vi "Duplicate Targets.vi"(9 "Array":T1[](array[typedef])) -> (2 "Duplicates found":bool)   [LabVIEW 2009]
uses:
  MixedMode/Messages/Target.ctl
  Data Access Objects/Metadata/LBCB Number.ctl
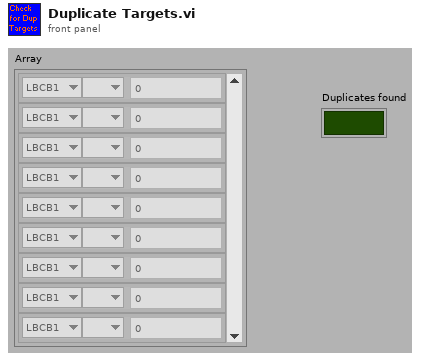
[diagram p1: front panel]
types:
  T1 = typedef "Target.ctl" = cluster{"LBCB Number":T2, "DOF Vectors":enum16{" ", "Dx", "Dy", "Dz", "Rx", "Ry", "Rz", "Fx", "Fy", "Fz", "Mx", "My", "Mz"}, "Amount":dbl}
  T2 = typedef "LBCB Number.ctl" = enum16{"LBCB1", "LBCB2"}
  T3 = enum16{" ", "Dx", "Dy", "Dz", "Rx", "Ry", "Rz", "Fx", "Fy", "Fz", "Mx", "My", "Mz"}
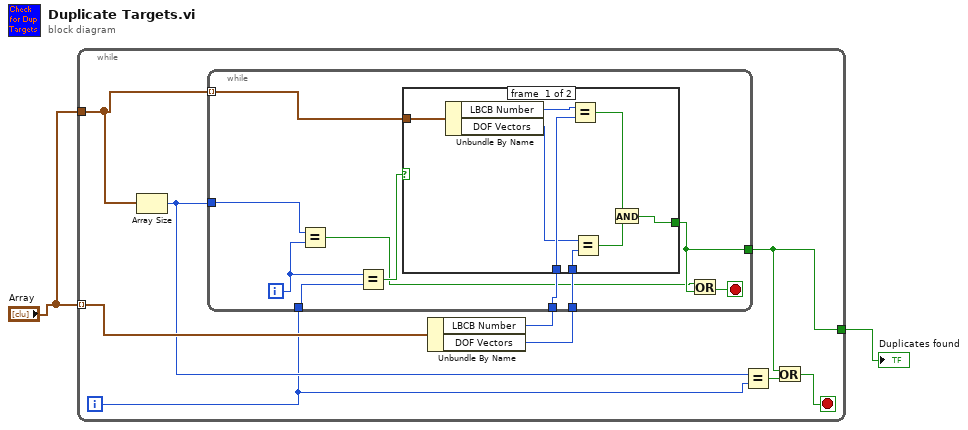
[diagram p0: block diagram]
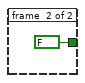
[diagram p2: hidden frame]
diagram:
  n1 = while {
    tunnel: "Array" -> [w9] mode=indexing
    tunnel: "Array" -> [w8]
    tunnel: [w4] -> w1
    i -> [w6]
    stop <- w3 stop-if-true
    n2 = Array Size(array=w8) -> (size(s)=w7:i32)
    n3 = Unbundle By Name(w9) -> ("LBCB Number"=w11:T2, "DOF Vectors"=w10:T3)
    n4 = while {
      tunnel: w11 -> [w21]
      tunnel: w10 -> [w20]
      tunnel: w8 -> [w19] mode=indexing
      tunnel: w6 -> [w18]
      tunnel: [w16] -> w4
      tunnel: w7 -> [w15]
      i -> [w14]
      stop <- w13 stop-if-true
      n5 = Equal?(x=w15, y=w14) -> (x = y?=w12:bool)
      n6 = Equal?(x=w14, y=w18) -> (x = y?=w17:bool)
      n7 = case shown="True" w17 {
        tunnel: w21 -> [w28 _]
        tunnel: w20 -> [w26 _]
        tunnel: [w23 FALSE] -> w16
        tunnel: w19 -> [w22 _]
        frame #0 {
          n8 = Unbundle By Name(w22) -> ("LBCB Number"=w29:T2, "DOF Vectors"=w27:T3)
          n9 = Equal?(x=w29, y=w28) -> (x = y?=w25:bool)
          n10 = Equal?(x=w27, y=w26) -> (x = y?=w24:bool)
          n11 = And(x=w25, y=w24) -> (x .and. y?=w23:bool)
        }
        frame #1 {
        }
      }
      n12 = Or(x=w12, y=w16) -> (x .or. y?=w13:bool)
    }
    n13 = Equal?(x=w7, y=w6) -> (x = y?=w5:bool)
    n14 = Or(x=w4, y=w5) -> (x .or. y?=w3:bool)
  }
  "Duplicates found" <- w1
